vi "Testing fgv.vi"(7 "Populate":bool, 8 "error in (no error)":errorcluster, 10 "test dir In":path, 11 "Testing? In":bool) -> (0 "error out":errorcluster, 2 "test dir":path, 3 "Testing?":bool)   [LabVIEW 2016]
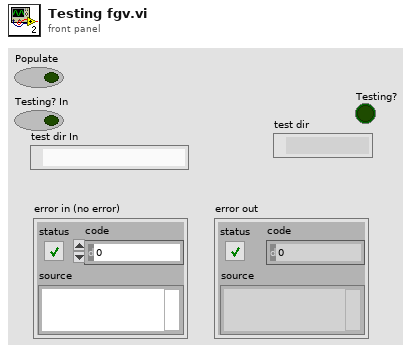
[diagram p1: front panel]
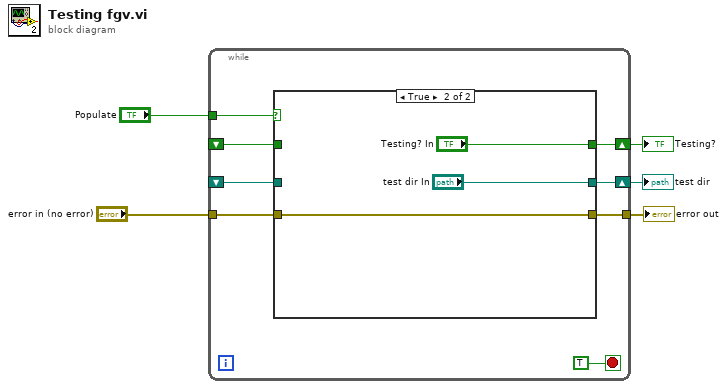
[diagram p0: block diagram]
diagram:
  n1 = while {
    tunnel: "Populate" -> [w12]
    tunnel: "error in (no error)" -> [w11]
    tunnel: [w10] -> w3
    shift-right: [w9] -> w1
    shift-left: _ -> [w8]
    shift-right: [w7] -> w2
    shift-left: _ -> [w6]
    stop <- TRUE stop-if-true
    n2 = case shown="True" w12 {
      tunnel: w11 -> [w16 w18]
      tunnel: [w16 w18] -> w10
      tunnel: [w14 "test dir In"] -> w9
      tunnel: w8 -> [w14 _]
      tunnel: [w15 "Testing? In"] -> w7
      tunnel: w6 -> [w15 _]
      frame False {
      }
      frame True {
      }
    }
  }
  "error out" <- w3
  "Testing?" <- w2
  "test dir" <- w1
